vi "write_fifo_resonance_ch0_ch1_FF_FB.vi"(5 "enable fly-back reversion?":bool, 6 "invert channels":bool[](array[boolean])=[FALSE, FALSE], 7 "fly-back?":bool, 8 "pixel finished?":bool, 10 "maximum bit depth":i8, 11 "integration cluster in":T1) -> (0 "FIFO overflow out":bool, 3 "integration cluster out":T1)   [LabVIEW 2010]
uses:
  integration_cluster.ctl
  <vilib>/rvi/DataTransferAndStorage/Container/XNode/niFpgaContainer.xnode
  <vilib>/rvi/DataTransferAndStorage/Container/Common/niFpgaContainerMethod.ctl
  <vilib>/rvi/DataTransferAndStorage/Container/Common/niFpgaTransferTypeControl.ctl
  <vilib>/rvi/Memory/Memory_Emulation/nirvimemoryEmulationManagerCache_GetValue.vi
  <vilib>/rvi/DataTransferAndStorage/Container/Common/niFpgaContainerGetUniqueNameForEmu.vi
  <vilib>/rvi/Memory/Memory_Emulation/nirvimemoryEmulationManagerCache_InsertValue.vi
  <vilib>/Utility/error.llb/Clear Errors.vi
  <vilib>/rvi/Memory/Memory_Emulation/nirvimemoryEmulationManagerCache_SetValue.vi
  <vilib>/rvi/interface/RandomDataEmulation/nirviRandomDataFPGAFIFO.vi
  <vilib>/rvi/interface/RandomDataEmulation/niFpgaRandomDataHandleErrors.vi
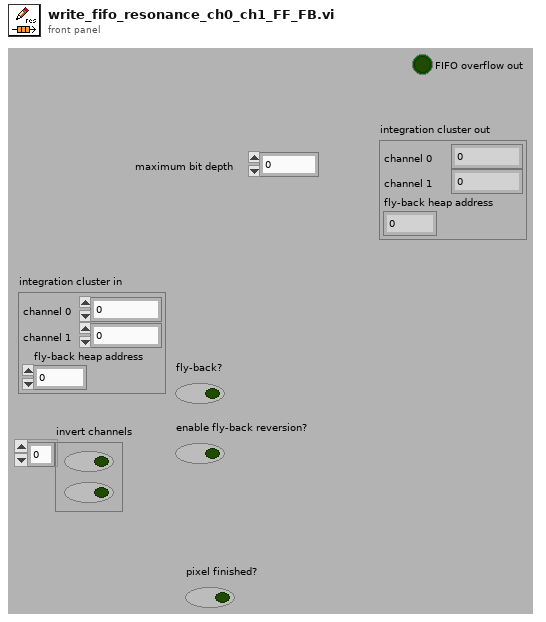
[diagram p1: front panel]
types:
  T1 = typedef "integration_cluster.ctl" = cluster{"channel 0":u32, "channel 1":u32, "fly-back heap address":u32}
  T2 = typedef "niFpgaContainerMethod.ctl" = enum16{"<none>", "write", "read", "clear", "getNumberOfElementsToWrite", "getNumberOfElementsToRead", "enable", "disable", "flushAndDisable", "getStreamState", "readA", "readB", "dramWrite", "dramWriteWithByteEnables", "dramRequestData", "dramRetrieveData"}
  T3 = typedef "niFpgaTransferTypeControl.ctl" = enum16{"Target-Scoped", "Host to Target - DMA", "Target to Host - DMA", "Peer to Peer Reader", "Peer to Peer Writer", "Bidirectional"}
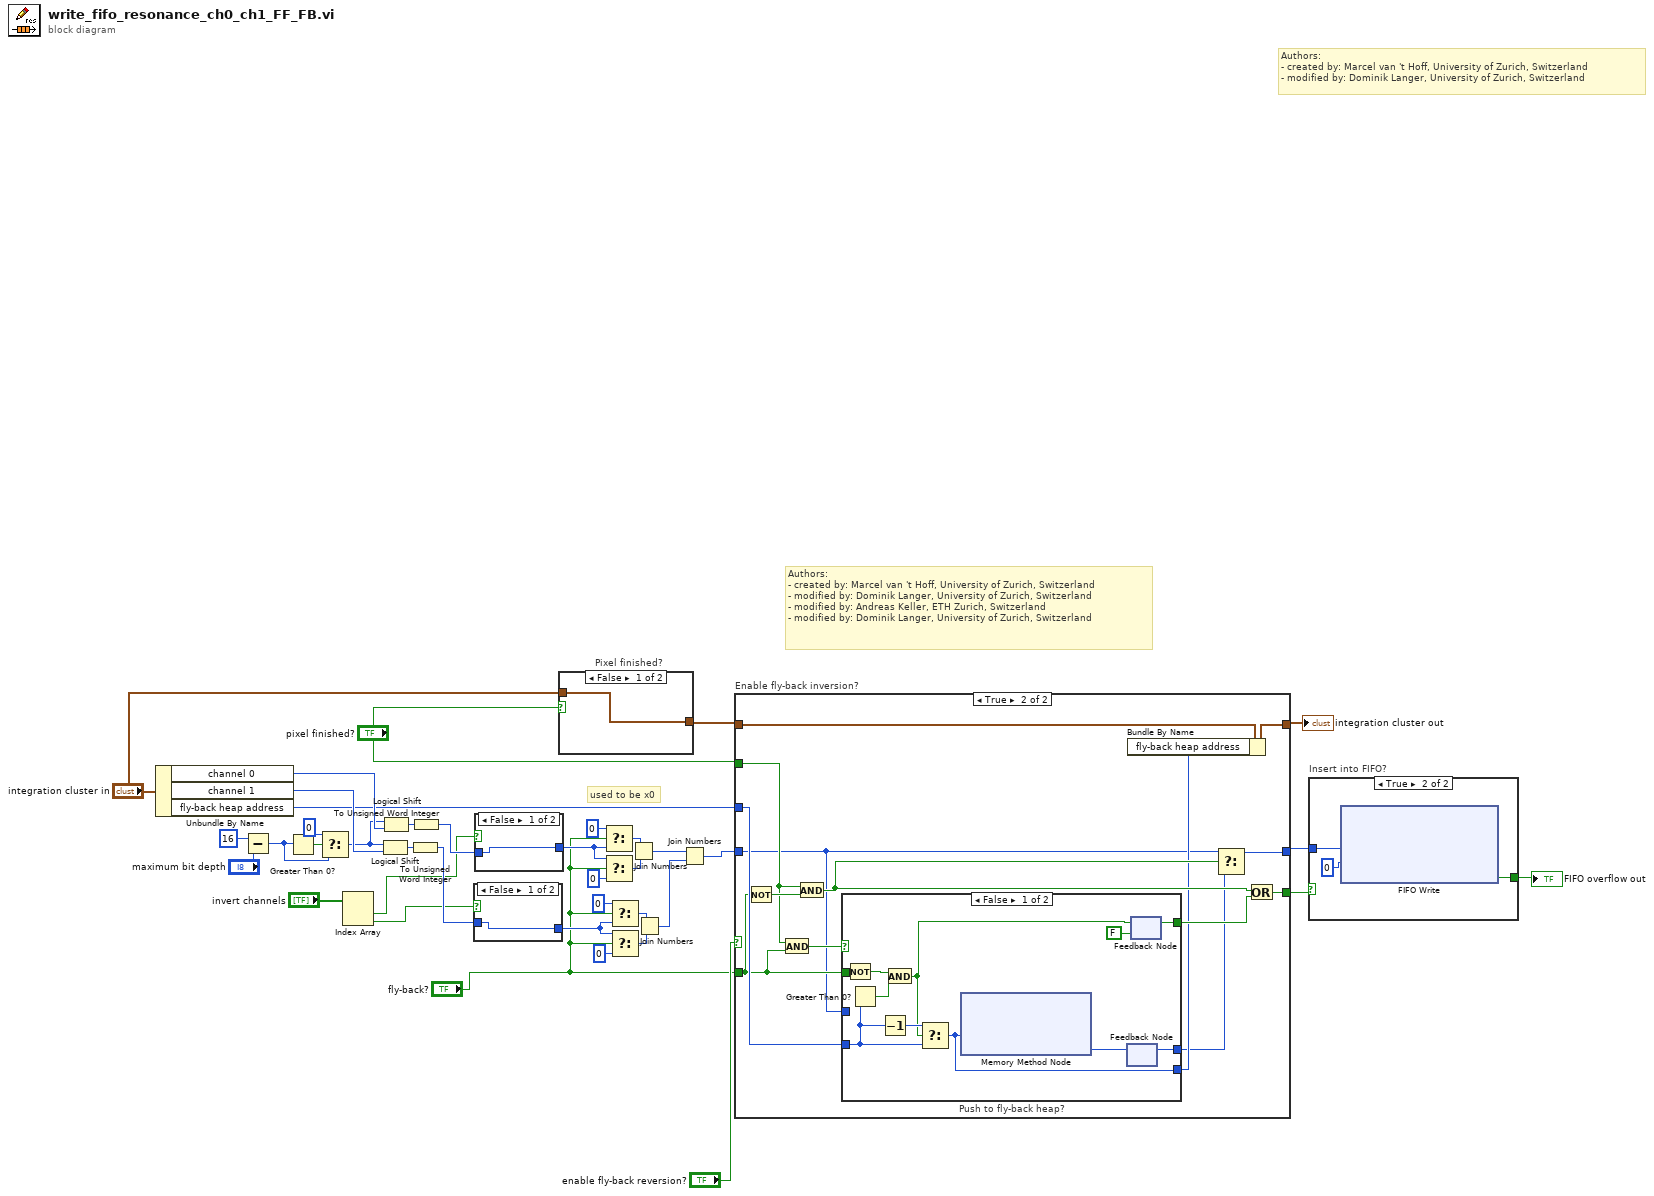
[diagram p0: block diagram]
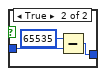
[diagram p2: hidden frame]
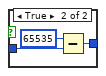
[diagram p3: hidden frame]
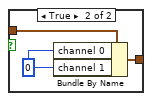
[diagram p4: hidden frame]
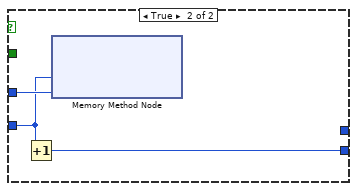
[diagram p6: hidden frame]
diagram:
  # "used to be x0"
  # "Authors: \n- created by: Marcel van 't Hoff, University of Zurich, Switzerland\n- modified by: Dominik Langer, University of Zurich, Switzerland\n- modified by: Andreas Keller, ETH Zurich, Switzerland\n- modified by: Dominik Langer, University of Zurich, Switzerland"
  # "Authors: \n- created by: Marcel van 't Hoff, University of Zurich, Switzerland\n- modified by: Dominik Langer, University of Zurich, Switzerland"
  n1 = Unbundle By Name("integration cluster in") -> ("channel 0"=w31:u32, "channel 1"=w32:u32, "fly-back heap address"=w25:u32)
  n2 = Subtract(x=i8 16, y="maximum bit depth") -> (x-y=w34:i8)
  n3 = Greater Than 0?(x=w34) -> (x > 0?=w33:bool)
  n4 = Select(t=i8 0 ("f"), s=w33, f=w34) -> (s? t:f=w30:i8)
  n5 = Index Array(array="invert channels") -> (element #1=w16:bool, element #2=w15:bool)  [unwired: 2 in]
  n6 = Logical Shift(y=w30, x=w32) -> (x << y=w29:u32)
  n7 = Logical Shift(y=w30, x=w31) -> (x << y=w28:u32)
  n8 = To Unsigned Word Integer(number=w29) -> (unsigned 16bit integer=w18:u16)
  n9 = To Unsigned Word Integer(number=w28) -> (unsigned 16bit integer=w19:u16)
  n10 = case shown="False" w15 {
    tunnel: [w39 w41] -> w5
    tunnel: w18 -> [w39 w40]
    frame False {
    }
    frame True {
      n11 = Subtract(x=u16 65535, y=w40) -> (x-y=w41:u16)
    }
  }
  n12 = case shown="False" w16 {
    tunnel: [w43 w45] -> w12
    tunnel: w19 -> [w43 w44]
    frame False {
    }
    frame True {
      n13 = Subtract(x=u16 65535, y=w44) -> (x-y=w45:u16)
    }
  }
  n14 = case "Pixel finished?" shown="False" "pixel finished?" {
    tunnel: "integration cluster in" -> [w47 w49]
    tunnel: [w47 w48] -> w22
    frame False {
    }
    frame True {
      w50 = u32 0 ("channel 1")
      n15 = Bundle By Name(cluster=w49, "channel 0"=w50, "channel 1"=w50) -> (w48:T1)
    }
  }
  n16 = Select(t=u16 0 ("x"), s="fly-back?", f=w12) -> (s? t:f=w14:u16)
  n17 = Select(t=w12, s="fly-back?", f=u16 0 ("x")) -> (s? t:f=w13:u16)
  n18 = Select(t=u16 0 ("x"), s="fly-back?", f=w5) -> (s? t:f=w9:u16)
  n19 = Select(t=w5, s="fly-back?", f=u16 0 ("x")) -> (s? t:f=w8:u16)
  n20 = Join Numbers(hi=w14, lo=w13) -> ((hi.lo)=w2:u32)
  n21 = Join Numbers(hi=w9, lo=w8) -> ((hi.lo)=w3:u32)
  n22 = Join Numbers(hi=w2, lo=w3) -> ((hi.lo)=w1:u64)
  n23 = case "Enable fly-back inversion?" shown="True" "enable fly-back reversion?" {
    tunnel: w25 -> [_ w67]
    tunnel: w1 -> [w53 w56]
    tunnel: [w53 w65] -> w27
    tunnel: "pixel finished?" -> [w52 w60]
    tunnel: [w52 w55] -> w24
    tunnel: "fly-back?" -> [_ w62]
    tunnel: w22 -> [w51 w59]
    tunnel: [w51 w57] -> w20
    frame False {
    }
    frame True {
      n24 = Not(x=w62) -> (.not. x?=w66:bool)
      n25 = And(x=w60, y=w62) -> (x .and. y?=w64:bool)
      n26 = And(x=w60, y=w66) -> (x .and. y?=w63:bool)
      n27 = case "Push to fly-back heap?" shown="False" w64 {
        tunnel: w56 -> [_ w207]
        tunnel: [w70 w206] -> w58
        tunnel: w67 -> [w72 w205]
        tunnel: w62 -> [w77 _]
        tunnel: [w74 _] -> w54
        tunnel: [w76 _] -> w61
        frame False {
          n28 = Not(x=w77) -> (.not. x?=w69:bool)
          n29 = Greater Than 0?(x=w72) -> (x > 0?=w78:bool)
          n30 = Decrement(x=w72) -> (x-1=w71:u32)
          n31 = And(x=w69, y=w78) -> (x .and. y?=w68:bool)
          n32 = Select(t=w71, s=w68, f=w72) -> (s? t:f=w70:u32)
          n33 = xnode ("Memory Method Node")("Address"=w70) -> ("Data"=w73:u32)  [unwired: 1 in, 1 out]
          n34 = feedback #1() -> (w74:u32)  [unwired: 1 in]
          n35 = feedback-in #1(w73) -> ()
          n36 = feedback #2(FALSE) -> (w76:bool)
          n37 = feedback-in #2(w68) -> ()
        }
        frame True {
          n38 = Increment(x=w205) -> (x+1=w206:u32)
          n39 = xnode ("Memory Method Node")("Address"=w205, "Data"=w207) -> ()  [unwired: 1 in, 1 out]
        }
      }
      n40 = Bundle By Name(cluster=w59, "fly-back heap address"=w58) -> (w57:T1)
      n41 = Select(t=w56, s=w63, f=w54) -> (s? t:f=w65:u64)
      n42 = Or(x=w63, y=w61) -> (x .or. y?=w55:bool)
    }
  }
  "integration cluster out" <- w20
  n43 = case "Insert into FIFO?" shown="True" w24 {
    tunnel: [_ w335] -> w37
    tunnel: w27 -> [_ w333]
    frame False {
    }
    frame True {
      n44 = xnode ("FIFO Write")("Element"=w333, "Timeout"=0) -> ("Timed Out?"=w335:bool)  [unwired: 1 in, 1 out]
    }
  }
  "FIFO overflow out" <- w37
